vi "Cluster API String to 1D Array(Splite Nested Cluster).vi"(8 "error in (no error)":errorcluster, 10 "trimmed string in":string) -> (0 "error out":errorcluster, 1 "Array of Strings":string[](array[string]))   [LabVIEW 2017, in "API String Arguments Support.lvlib"]
uses:
  API String Arguments Support.lvlib
  <userlib>/_NEVSTOP/Communicable State Machine(CSM)/Communicable State Machine.lvlib
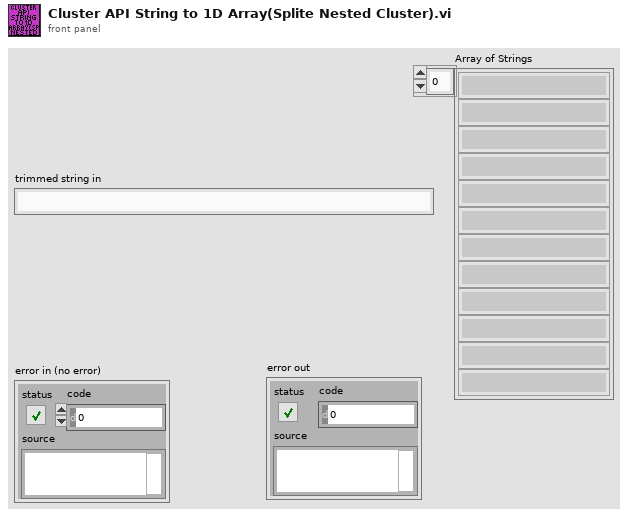
[diagram p1: front panel]
types:
  T1 = enum16{"0x2829 - ()", "0x5B5D - []", "0x7B7D - {}"}
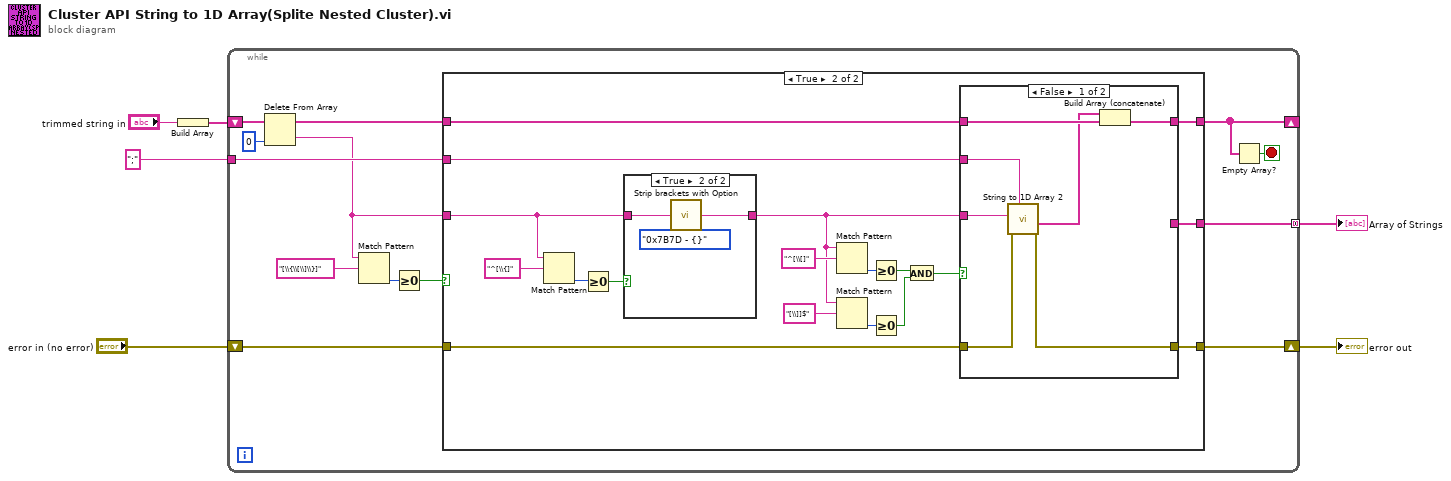
[diagram p0: block diagram]
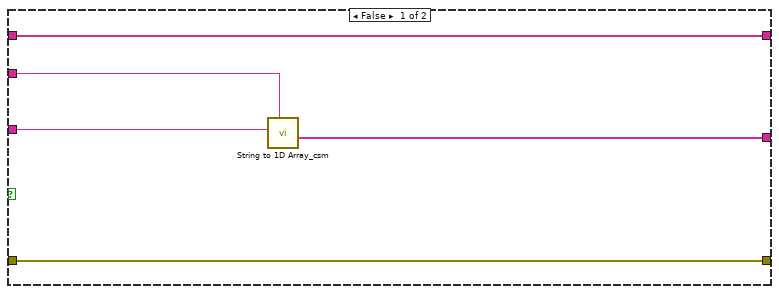
[diagram p2: hidden frame]
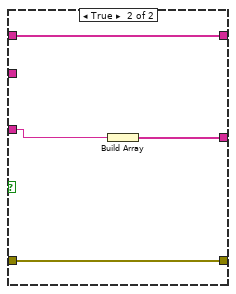
[diagram p3: hidden frame]
diagram:
  n1 = Build Array("trimmed string in") -> (w1:string[])
  n2 = while {
    tunnel: ";" ("delimiter") -> [w19]
    tunnel: [w14] -> w3 mode=concatenating
    shift-right: [w18] -> w5
    shift-left: "error in (no error)" -> [w17]
    shift-right: [w8] -> _
    shift-left: w1 -> [w13]
    stop <- w9 stop-if-true
    n3 = Delete From Array(array=w13, index=0) -> (deleted portion=w11:string, array with subset deleted=w10:string[])  [unwired: 1 in]
    n4 = Match Pattern(string=w11, regular expression="[\\{\\[\\]\\}]") -> (offset past match=w15:i32)  [unwired: 1 in, 3 out]
    n5 = Greater Or Equal To 0?(x=w15) -> (x >= 0?=w16:bool)
    n6 = case shown="True" w16 {
      tunnel: [w24 w25] -> w14
      tunnel: w11 -> [w23 w36]
      tunnel: w17 -> [w22 w42]
      tunnel: [w22 w41] -> w18
      tunnel: w19 -> [w21 w40]
      tunnel: w10 -> [w20 w39]
      tunnel: [w20 w38] -> w8
      frame False {
        n7 = call <userlib>:"String to 1D Array_csm.vi"("delimiter (Tab)"=w21, "string"=w23) -> ("Array of Strings"=w24:string[])  [unwired: 9 in]
      }
      frame True {
        n8 = Match Pattern(string=w36, regular expression="^[\\{]") -> (offset past match=w35:i32)  [unwired: 1 in, 3 out]
        n9 = Greater Or Equal To 0?(x=w35) -> (x >= 0?=w34:bool)
        n10 = case shown="True" w34 {
          tunnel: w36 -> [w54 w57]
          tunnel: [w54 w55] -> w31
          frame False {
          }
          frame True {
            n11 = call "Strip brackets with Option.vi"("TYPE"=T1."0x7B7D - {}", "trimmed string in"=w57) -> ("trimmed string out"=w55:string)  [unwired: 2 in]
          }
        }
        n12 = Match Pattern(string=w31, regular expression="^[\\[]") -> (offset past match=w30:i32)  [unwired: 1 in, 3 out]
        n13 = Match Pattern(string=w31, regular expression="[\\]]$") -> (offset past match=w28:i32)  [unwired: 1 in, 3 out]
        n14 = Greater Or Equal To 0?(x=w30) -> (x >= 0?=w29:bool)
        n15 = Greater Or Equal To 0?(x=w28) -> (x >= 0?=w27:bool)
        n16 = And(x=w29, y=w27) -> (x .and. y?=w26:bool)
        n17 = case shown="False" w26 {
          tunnel: w42 -> [w49 w51]
          tunnel: [w48 w51] -> w41
          tunnel: w40 -> [w47 _]
          tunnel: w39 -> [w46 w53]
          tunnel: [w45 w53] -> w38
          tunnel: w31 -> [w43 w52]
          tunnel: [_ w50] -> w25
          frame False {
            n18 = call "String to 1D Array 2.vi"("delimiter (,)"=w47, "Error in"=w49, "string"=w43) -> ("Error out"=w48:errorcluster, "Array of Strings"=w44:string[])  [unwired: 7 in]
            n19 = Build Array (concatenate)(w44, w46) -> (w45:string[])
          }
          frame True {
            n20 = Build Array(w52) -> (w50:string[])
          }
        }
      }
    }
    n21 = Empty Array?(array=w8) -> (empty?=w9:bool)
  }
  "error out" <- w5
  "Array of Strings" <- w3
